vi "Autotest_Instr.vi"(8 "error in (no error)":errorcluster caption="entrée d'erreur (pas d'erreur)", 11 "Class Relay_Board en entrée":refnum<class "Class Instrument UART.lvclass">) -> (0 "error out":errorcluster caption="sortie d'erreur", 3 "Class Relay_Board en Sortie":refnum<class "Class Instrument UART.lvclass">)   [LabVIEW 2020, in "Library Instrument & Equipement.lvlib" / "Library Instruments.lvlib" / "Class Instrument UART.lvclass"]
uses:
  Class Instrument UART.lvclass
  C:/Users/ngarcin/OneDrive - Altyor/Standard TB/Class/Instrument/Instrument (Default)/Class Instrument (Default).lvclass
  Class Instrument UART.lvclass/Class Instrument UART.ctl
  Instrument (Default)/Class Instrument (Default).lvclass
  UART/UART (Default)/Class UART (Default).lvclass
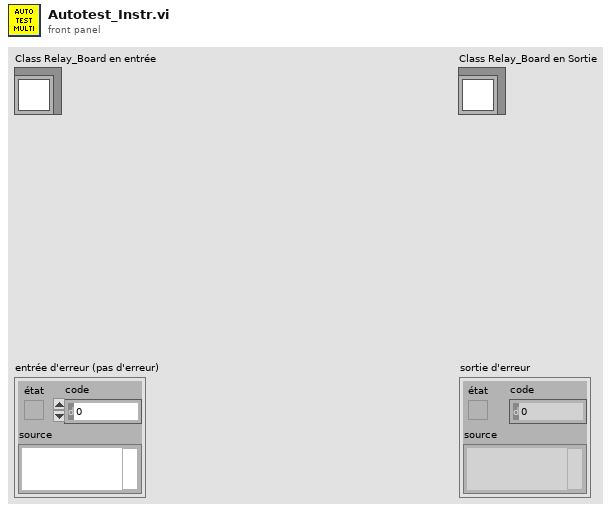
[diagram p1: front panel]
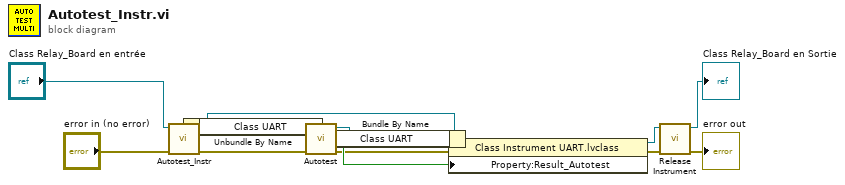
[diagram p0: block diagram]
diagram:
  n1 = call-parent "Autotest_Instr.vi"("error in (no error)"="error in (no error)", "Class Instrument (Default) en entrée"="Class Relay_Board en entrée") -> ("error out"=w5:errorcluster, "Class Instrument (Default) en sortie"=w11:refnum<class "Class Instrument UART.lvclass">)  [unwired: 8 in]
  n2 = Unbundle By Name(w11) -> ("Class UART"=w1:refnum<class "Class UART (Default).lvclass">)
  n3 = call-dynamic "Autotest.vi"("error in (no error)"=w5, "Class UART (Default) en entrée"=w1) -> ("error out"=w3:errorcluster, "Autotest Ok"=w4:bool, "Class UART (Default) en sortie"=w2:refnum<class "Class UART (Default).lvclass">)  [unwired: 7 in]
  n4 = Bundle By Name(cluster=w11, "Class UART"=w2) -> (w10:refnum<class "Class Instrument UART.lvclass">)
  n5 = property class="Class Instrument UART.lvclass"(reference=w10, error in=w3, "Property:Result_Autotest"=w4) -> (reference out=w7:refnum<class "Class Instrument UART.lvclass">, error out=w9:errorcluster)
  n6 = call-dynamic "Release Instrument.vi"("error in (no error)"=w9, "Class Instrument (Default) en entrée"=w7) -> ("error out"=→"error out":errorcluster, "Class Instrument (Default) en sortie"=→"Class Relay_Board en Sortie":refnum<class "Class Instrument UART.lvclass">)  [unwired: 8 in]
